vi "Configure Report Channel.vi"(0 "VISA resource name":refnum<visa-resource-name>, 1 "Sum Scale (0: Off)":i32(ring) items=["Off", "/sec", "/min", "/hour", "/day"], 5 "Report Channel Number (1)":i32=1 min=1 max=60 step=1, 7 "Channel Type (0: Off)":i32(ring) items=["Off", "IO", "Math", "Communication"], 9 "Channel (0001)":string="0001", 11 "error in (no error)":errorcluster) -> (4 "VISA resource name out":refnum<visa-resource-name>, 15 "error out":errorcluster)   [LabVIEW 2020, in "Yokogawa GX Series.lvlib"]
doc: "Sets the type of data to record.\n\nCommand: SMemory"
uses:
  <instrlib>/Yokogawa GX Series/Yokogawa GX Series.lvlib
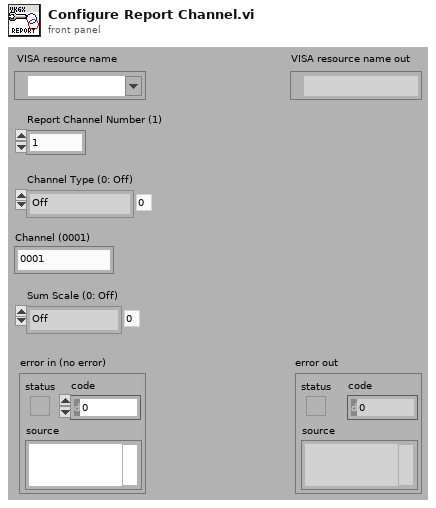
[diagram p1: front panel]
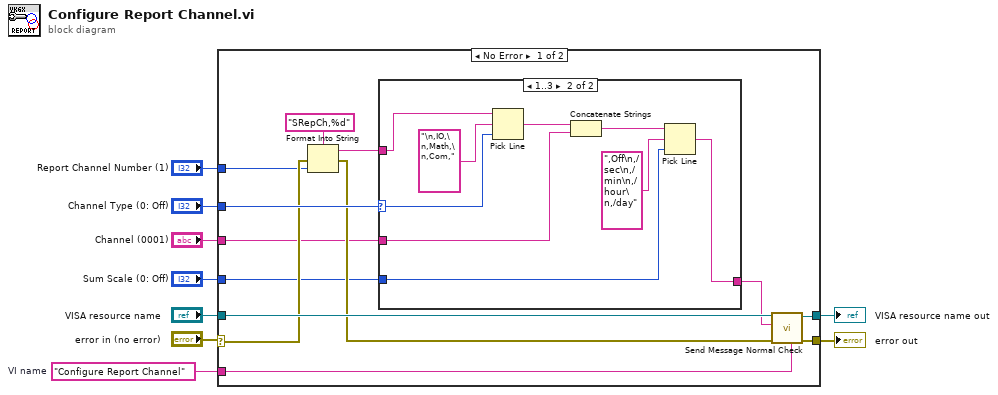
[diagram p0: block diagram]
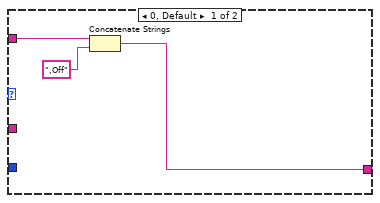
[diagram p2: hidden frame]
diagram:
  w8 = "Configure Report Channel"  # VI name
  n1 = case shown="No Error" "error in (no error)" {
    selector: "error in (no error)" -> [w15 w35]
    tunnel: "VISA resource name" -> [w22 w36]
    tunnel: w8 -> [w19 _]
    tunnel: [w21 w36] -> w7
    tunnel: [w20 w35] -> w6
    tunnel: "Channel Type (0: Off)" -> [w17 _]
    tunnel: "Report Channel Number (1)" -> [w13 _]
    tunnel: "Channel (0001)" -> [w11 _]
    tunnel: "Sum Scale (0: Off)" -> [w10 _]
    frame No Error {
      n2 = Format Into String(format string="SRepCh,%d", error in=w15, w13) -> (resulting string=w12:string, error out=w14:errorcluster)  [unwired: 1 in]
      n3 = case shown="1..3" w17 {
        selector: w17 -> [_ w34]
        tunnel: [w25 w26] -> w18
        tunnel: w12 -> [w24 w33]
        tunnel: w11 -> [_ w30]
        tunnel: w10 -> [_ w27]
        frame 0, Default {
          n4 = Concatenate Strings(w24, ",Off") -> (w25:string)
        }
        frame 1..3 {
          n5 = Pick Line(string ("")=w33, multi-line string="\n,IO,\n,Math,\n,Com,", line index=w34) -> (output string=w31:string)
          n6 = Concatenate Strings(w31, w30) -> (w29:string)
          n7 = Pick Line(string ("")=w29, multi-line string=",Off\n,/sec\n,/min\n,/hour\n,/day", line index=w27) -> (output string=w26:string)
        }
      }
      n8 = call <instrlib>:"Send Message Normal Check.vi"("Source (\"\")"=w19, "error in (no error)"=w14, "Send Message (\"\")"=w18, "VISA resource name"=w22) -> ("error out"=w20:errorcluster, "VISA resource name out"=w21:refnum<visa-resource-name>)  [unwired: 2 in, 4 out]
    }
    frame Error {
    }
  }
  "error out" <- w6
  "VISA resource name out" <- w7
